vi "Init Tips.vi"(8 "error in (no error)":errorcluster, 11 "[V] Login in":refnum<class "[V] Login.lvclass">) -> (0 "error out":errorcluster, 3 "[V] Login out":refnum<class "[V] Login.lvclass">)   [LabVIEW 2020, in "[V] Login.lvlib" / "[V] Login.lvclass"]
uses:
  [V] Login.lvclass
  [V] Login.lvclass/[V] Login.ctl
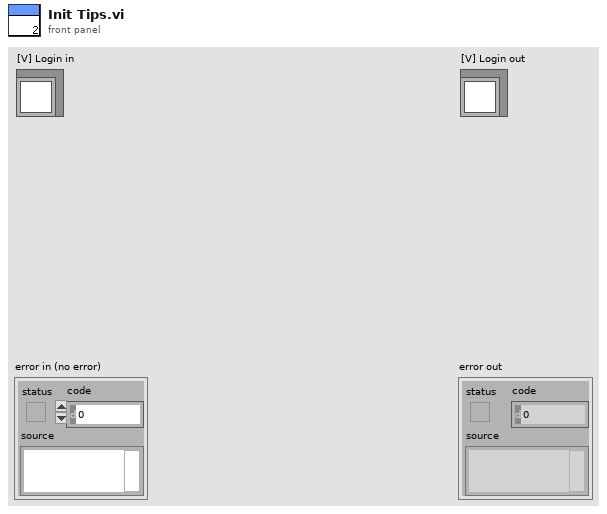
[diagram p1: front panel]
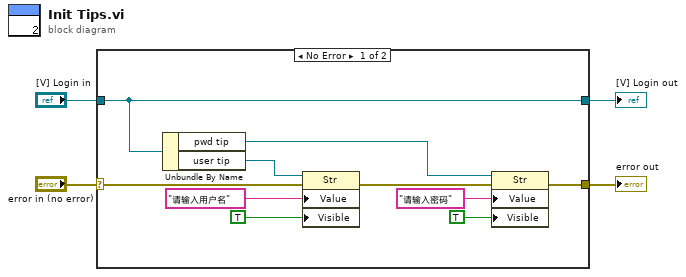
[diagram p0: block diagram]
diagram:
  n1 = case shown="No Error" "error in (no error)" {
    selector: "error in (no error)" -> [w13 w16]
    tunnel: [w5 w16] -> w3
    tunnel: [w14 w15] -> w1
    tunnel: "[V] Login in" -> [w14 w15]
    frame No Error {
      n2 = Unbundle By Name(w14) -> ("pwd tip"=w8:refnum<vi>, "user tip"=w12:refnum<vi>)
      n3 = property class="Str"(reference=w12, error in=w13, "Value"="请输入用户名", "Visible"=TRUE) -> (error out=w9:errorcluster)  [unwired: 1 out]
      n4 = property class="Str"(reference=w8, error in=w9, "Value"="请输入密码", "Visible"=TRUE) -> (error out=w5:errorcluster)  [unwired: 1 out]
    }
    frame Error {
    }
  }
  "error out" <- w3
  "[V] Login out" <- w1
